vi "SHA384.vi"(8 "error in (no error)":errorcluster, 11 "Data in":u8[](array[numeric])) -> (0 "error out":errorcluster, 3 "SHA384 Hash":u8[](array[numeric]))   [LabVIEW 2021, in "dotNET Crypto Hashing.lvlib"]
doc: "Computes the SHA384 hash of the message using .NET CNG API."
uses:
  dotNET Crypto Hashing.lvlib
  System.Core
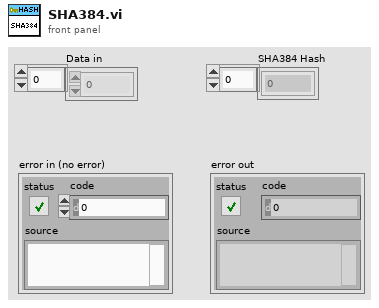
[diagram p1: front panel]
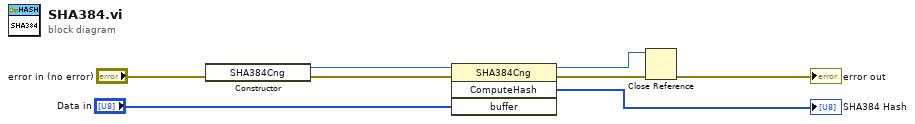
[diagram p0: block diagram]
diagram:
  n1 = constructor class="SHA384Cng"(error in="error in (no error)") -> (reference out=w6:refnum<k24>, error out=w5:errorcluster)  [unwired: 2 in, 1 out]
  n2 = invoke class="SHA384Cng" method="ComputeHash"(reference=w6, error in=w5, "buffer"="Data in") -> (reference out=w4:refnum<k24>, error out=w3:errorcluster, "ComputeHash"=→"SHA384 Hash":u8[])  [unwired: 1 in, 1 out]
  n3 = Close Reference(reference=w4, error in (no error)=w3) -> (error out=→"error out":errorcluster)
